vi "HighEnd-RT.vi"() -> ()   [LabVIEW 2016]
uses:
  <vilib>/rvi/interface/nirviReadWriteControl/nirviReadWriteControl.xnode
  <vilib>/rvi/interface/nirviOpenFPGA/nirviOpenFPGA.xnode
  Common-Control/Beamline sections/High Energy End/HighEnd-FPGA.vi
  Glassman Control.ctl
  GP307 cluster.ctl
  NiFpgaLv.dll
  <vilib>/Utility/error.llb/Error Cluster From Error Code.vi
  <vilib>/rvi/errors/niLvFpgaAdjustHostInterfaceError.vi
  Controls/GV states.ctl
  Controls/Faraday cup states.ctl
  <vilib>/NI_Real-Time Target Support.lvlib
  FPGA Bitfiles/PRIMEControl2017_FPGATarget3_HighEnd-FPGA_o8tZdM+PVqs.lvbitx
  <vilib>/FPGAPlugInAG/cRIO-9074/niLvFpga_Open_cRIO-9074.vi
panel:
  in  "Tab Control":T1(tab)
  out "ES Quad A+ I readback":fxp<+/-,16,5>
  out "ES Quad A+ V readback":fxp<+/-,16,5>
  out "ES Quad A- I readback":fxp<+/-,16,5>
  out "ES Quad A- V readback":fxp<+/-,16,5>
  out "ES Quad B+ I readback":fxp<+/-,16,5>
  out "Y1- Steerer V set":dbl
  out "Y2+ Steerer V set":dbl
  out "Y2- Steerer V set":dbl
  out "ES Quad A V set":dbl
  out "ES Quad B V set":dbl
  out "ES Quad B+ V readback":fxp<+/-,16,5>
  out "ES Quad B- I readback":fxp<+/-,16,5>
  out "ES Quad B- V readback":fxp<+/-,16,5>
  out "X+ Steerer I readback":fxp<+/-,26,5>
  out "X+ Steerer V readback":fxp<+/-,26,7>
  out "X- Steerer  I readback":fxp<+/-,16,5>
  out "X- Steerer V readback":fxp<+/-,16,5>
  out "Y1+ Steerer  I readback":fxp<+/-,16,5>
  out "Y1+ Steerer V readback":fxp<+/-,16,5>
  out "Y1- Steerer  I readback":fxp<+/-,16,5>
  out "Y1- Steerer V readback":fxp<+/-,16,5>
  out "Y2+ Steerer  I readback":fxp<+/-,16,5>
  out "Y2+ Steerer V readback":fxp<+/-,16,5>
  out "Y2- Steerer  I readback":fxp<+/-,16,5>
  out "Y2- Steerer V readback":fxp<+/-,16,5>
  out "X+ Steerer V set":dbl
  out "X- Steerer V set":dbl
  out "X- Steerer HV Enable":bool
  out "Y1+ Steerer V set":dbl
  out "Y1+ Steerer HV Enable":bool
  out "Y1- Steerer HV Enable":bool
  out "Y2+ Steerer HV Enable":bool
  out "Y2- Steerer HV Enable":bool
  out "ES Quad A HV Enable":bool
  out "ES Quad B HV Enable":bool
  out "X+ Steerer HV Enable":bool
  out "Analyzer Object Vac cluster":T2
  out "Tank Exit Vac cluster":T2
  out "Vac readback loop error":errorcluster
  out "Ion gauge 1":u8[](array[numeric])
  out "Convectron 1":u8[](array[numeric])
  out "Ion gauge 2":u8[](array[numeric])
  out "Convectron 2":u8[](array[numeric])
  out "Ion gauge 3":u8[](array[numeric])
  out "Convectron 4":u8[](array[numeric])
  out "Ion gauge 4":u8[](array[numeric])
  out "Convectron 4":u8[](array[numeric])
  out "High End waist interlock bypass":bool
  out "Tank Exit Vac Interlock":bool
  out "High End Waist Vac Interlock":bool
  out "Analyzer Image Vac Interlock":bool
  out "Tank Exit interlock bypass":bool
  out "Analyzer Image Interlock Bypass":bool
  out "Tank Exit FC Actuator":bool
  out "Cryo Pump GV Actuator":bool
  out "Beamline GV Actuator":bool
  out "Beamline Fast GV actuator":bool
  out "Turbo GV actuator":bool
  out "Beamline Fast GV status":T3
  out "Beamline Fast GV Position":T4
  out "Turbo GV status":T3
  out "Turbo GV Position":T4
  out "Beamline GV status":T3
  out "Beamline GV Position":T4
  out "Tank Exit FC Status":T5
  out "Tank Exit FC Position":cluster{"IN sensor":bool, "OUT sensor":bool}
  out "Cryo Pump GV status":T3
  out "Cryo Pump GV Position":T4
  out "HV readback loop error":errorcluster
  out "Interlock loop error":errorcluster
  out "Actuator Sensor loop error":errorcluster
  out "HV control loop error":errorcluster
  out "Error Reporter":errorcluster
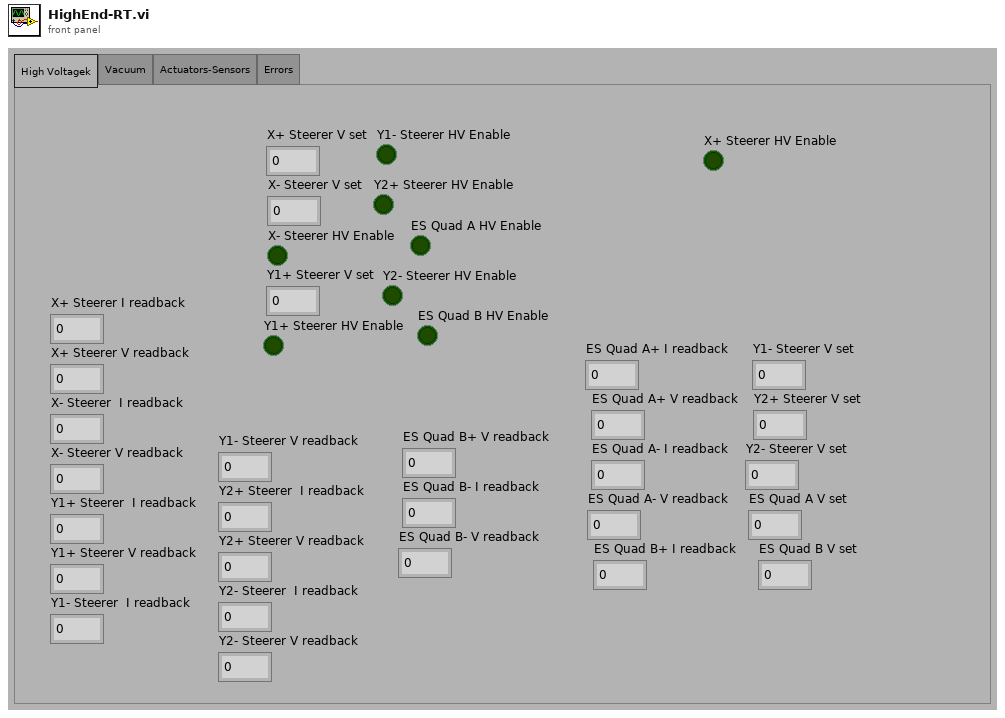
[diagram p1: front panel]
types:
  T1 = enum32{"High Voltagek", "Vacuum", "Actuators-Sensors", "Errors"}
  T2 = cluster{"Ion gauge 1":string, "Convectron  Gauge 1 ":string, "Ion Gauge 2":string, "Convectrom Gauge 2":string}
  T3 = typedef "GV states.ctl" = enum16{"status unclear", "closed", "open"}
  T4 = cluster{"OPEN sensor":bool, "Closed sensor":bool}
  T5 = typedef "Faraday cup states.ctl" = enum16{"FC status unclear", "FC in", "FC out"}
  T6 = typedef "Glassman Control.ctl" = cluster{"V-program":fxp<+/-,16,5>, "HV Enable":bool}
  T7 = typedef "GP307 cluster.ctl" = cluster{"Ion gauge 1":string, "Convectron  Gauge 1 ":string, "Ion Gauge 2":string, "Convectrom Gauge 2":string}
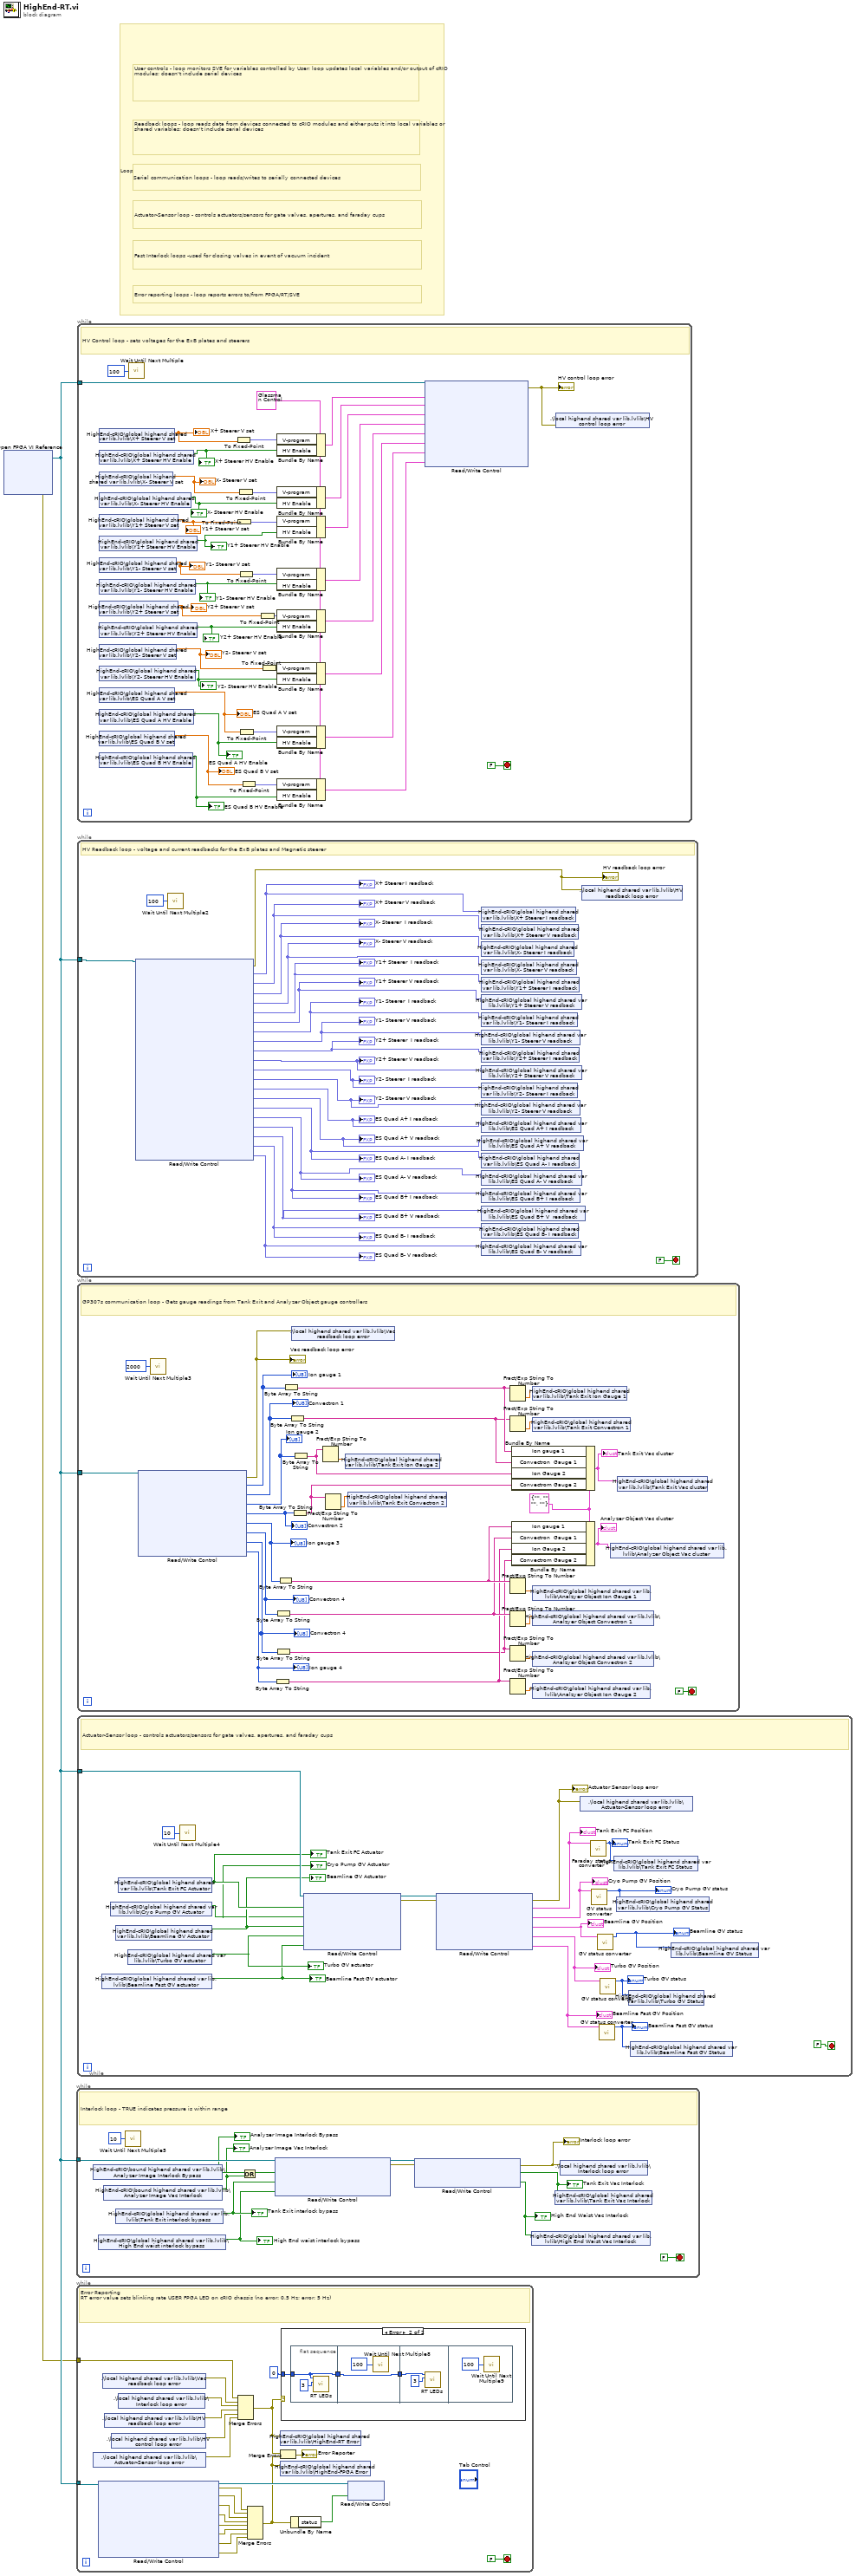
[diagram p0: block diagram]
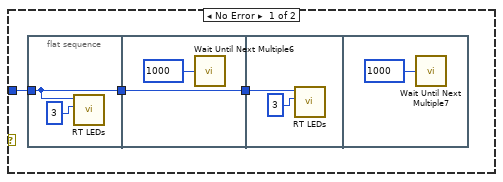
[diagram p2: hidden frame]
diagram:
  # "Serial communication loops - loop reads/writes to serially connected devices"
  # "Actuator-Sensor loop - controls actuators/sensors for gate valves, apertures, and faraday cups"
  # "Fast Interlock loops -used for closing valves in event of vacuum incident"
  # "Error reporting loops - loop reports errors to/from FPGA/RT/SVE"
  # "Readback loops - loop reads data from devices connected to cRIO modules and either puts it into local variables or shared variables; doesn't include serial devices"
  # "User controls - loop monitors SVE for variables controlled by User; loop updates local variables and/or output of cRIO modules; doesn't include serial devices"
  # "Loop legend - loops are color coded by responsibility"
  n1 = xnode "Open FPGA VI Reference"() -> ("FPGA VI Reference Out"=w2:refnum<k20>, "error out"=w1:errorcluster)  [unwired: 2 in]
  n2 = while {
    tunnel: w2 -> [w15]
    stop <- FALSE stop-if-true
    # "Interlock loop - TRUE indicates pressure is within range"
    n3 = shared-variable "HighEnd-cRIO\\bound highend shared var lib.lvlib\\Analyzer Image Interlock Bypass"() -> (w11:bool)  [unwired: 1 in, 1 out]
    "Analyzer Image Interlock Bypass" <- w11
    n4 = shared-variable "HighEnd-cRIO\\global highend shared var lib.lvlib\\High End waist interlock bypass"() -> (w6:bool)  [unwired: 1 in, 1 out]
    "High End waist interlock bypass" <- w6
    n5 = shared-variable "HighEnd-cRIO\\bound highend shared var lib.lvlib\\Analyzer Image Vac Interlock"() -> (w9:bool)  [unwired: 1 in, 1 out]
    "Analyzer Image Vac Interlock" <- w9
    n6 = shared-variable "HighEnd-cRIO\\global highend shared var lib.lvlib\\Tank Exit interlock bypass"() -> (w7:bool)  [unwired: 1 in, 1 out]
    "Tank Exit interlock bypass" <- w7
    n7 = call "Wait Until Next Multiple5"("Count(mSec)"=u32 10 ("millisecond multiple")) -> ()  [unwired: 1 out]
    n8 = Or(x=w11, y=w9) -> (x .or. y?=w10:bool)
    n9 = xnode "Read/Write Control"("FPGA VI Reference In"=w15, "Analyzer Image Vac Interlock"=w10, "Tank Exit interlock bypass"=w7, "High End waist interlock bypass"=w6) -> ("FPGA VI Reference Out"=w13:refnum<k20>, "error out"=w12:errorcluster)  [unwired: 1 in]
    n10 = xnode "Read/Write Control"("FPGA VI Reference In"=w13, "error in"=w12) -> ("error out"=w8:errorcluster, "Tank Exit Vac Interlock"=w5:bool, "High End Waist Vac Interlock"=w4:bool)  [unwired: 1 out]
    "Interlock loop error" <- w8
    "Tank Exit Vac Interlock" <- w5
    "High End Waist Vac Interlock" <- w4
    n11 = shared-variable "HighEnd-cRIO\\global highend shared var lib.lvlib\\High End Waist Vac Interlock"(w4) -> ()  [unwired: 1 in, 1 out]
    n12 = shared-variable "HighEnd-cRIO\\global highend shared var lib.lvlib\\Tank Exit Vac Interlock"(w5) -> ()  [unwired: 1 in, 1 out]
    n13 = shared-variable ".\\local highend shared var lib.lvlib\\Interlock loop error"(w8) -> ()  [unwired: 1 in, 1 out]
  }
  n14 = while {
    tunnel: w2 -> [w36]
    tunnel: w1 -> [w20]
    stop <- FALSE stop-if-true
    # "Error Reporting\nRT error value sets blinking rate USER FPGA LED on cRIO chassis (no error: 0.5 Hz; error: 5 Hz)"
    n15 = shared-variable ".\\local highend shared var lib.lvlib\\Actuator-Sensor loop error"() -> (w25:errorcluster)  [unwired: 1 in, 1 out]
    n16 = xnode "Read/Write Control"("FPGA VI Reference In"=w36) -> ("FPGA VI Reference Out"=w35:refnum<k20>, "error out"=w34:errorcluster, "GV Interlock loop error"=w33:errorcluster, "Actuator loop error"=w32:errorcluster, "Tank Exit Vac Gauge error"=w31:errorcluster, "Analyzer Obj Vac Gauge error"=w30:errorcluster, "Steerer HV readback loop error"=w29:errorcluster, "ES Quad HV readback loop error"=w28:errorcluster, "HV control loop error"=w27:errorcluster)  [unwired: 1 in]
    n17 = shared-variable ".\\local highend shared var lib.lvlib\\Vac readback loop error"() -> (w21:errorcluster)  [unwired: 1 in, 1 out]
    n18 = shared-variable ".\\local highend shared var lib.lvlib\\HV readback loop error"() -> (w23:errorcluster)  [unwired: 1 in, 1 out]
    n19 = shared-variable ".\\local highend shared var lib.lvlib\\HV control loop error"() -> (w24:errorcluster)  [unwired: 1 in, 1 out]
    n20 = shared-variable ".\\local highend shared var lib.lvlib\\Interlock loop error"() -> (w22:errorcluster)  [unwired: 1 in, 1 out]
    n21 = Merge Errors(w20, w21, w22, w23, w24, w25) -> (w16:errorcluster)
    n22 = Merge Errors(w34, w33, w32, w31, w30, w29, w28, w27) -> (w18:errorcluster)
    n23 = shared-variable "HighEnd-cRIO\\global highend shared var lib.lvlib\\HighEnd-RT Error"(w16) -> ()  [unwired: 1 in, 1 out]
    n24 = Merge Errors(w16, w18) -> (→"Error Reporter":errorcluster)
    n25 = shared-variable "HighEnd-cRIO\\global highend shared var lib.lvlib\\HighEnd-FPGA Error"(w18) -> ()  [unwired: 1 in, 1 out]
    n26 = case shown="Error" w16 {
      tunnel: 0 -> [w40 w48]
      frame No Error {
        n27 = flat-sequence {
          tunnel: w40 -> [w41]
          tunnel: [w41] -> w38
          tunnel: [w43] -> w39
          tunnel: w38 -> [w43]
          tunnel: w39 -> [w45]
          frame #0 {
            n28 = call <vilib>:"RT LEDs.vi"("State"=3, "LED Num"=w41) -> ()  [unwired: 4 in, 2 out]
          }
          frame #1 {
            n29 = call "Wait Until Next Multiple6"("Count(mSec)"=u16 1000) -> ()  [unwired: 1 out]
          }
          frame #2 {
            n30 = call <vilib>:"RT LEDs.vi"("State"=3, "LED Num"=w45) -> ()  [unwired: 4 in, 2 out]
          }
          frame #3 {
            n31 = call "Wait Until Next Multiple7"("Count(mSec)"=u16 1000) -> ()  [unwired: 1 out]
          }
        }
      }
      frame Error {
        n32 = flat-sequence {
          tunnel: [w51] -> w50
          tunnel: w48 -> [w51]
          tunnel: w50 -> [w53]
          tunnel: [w53] -> w49
          tunnel: w49 -> [w55]
          frame #0 {
            n33 = call <vilib>:"RT LEDs.vi"("State"=3, "LED Num"=w51) -> ()  [unwired: 4 in, 2 out]
          }
          frame #1 {
            n34 = call "Wait Until Next Multiple8"("Count(mSec)"=u16 100) -> ()  [unwired: 1 out]
          }
          frame #2 {
            n35 = call <vilib>:"RT LEDs.vi"("State"=3, "LED Num"=w55) -> ()  [unwired: 4 in, 2 out]
          }
          frame #3 {
            n36 = call "Wait Until Next Multiple9"("Count(mSec)"=u16 100) -> ()  [unwired: 1 out]
          }
        }
      }
    }
    n37 = Unbundle By Name(w18) -> ("status"=w37:bool)
    n38 = xnode "Read/Write Control"("FPGA VI Reference In"=w35, "RT error"=w37) -> ()  [unwired: 1 in, 2 out]
  }
  n39 = while {
    tunnel: w2 -> [w94]
    stop <- FALSE stop-if-true
    w69 = T6 {"V-program"=0.0, "HV Enable"=FALSE} ("Glassman Control")
    # "HV Control loop - sets voltages for the ExB plates and steerers"
    n40 = shared-variable "HighEnd-cRIO\\global highend shared var lib.lvlib\\X+ Steerer V set"() -> (w90:dbl)  [unwired: 1 in, 1 out]
    "X+ Steerer V set" <- w90
    n41 = shared-variable "HighEnd-cRIO\\global highend shared var lib.lvlib\\X+ Steerer HV Enable"() -> (w89:bool)  [unwired: 1 in, 1 out]
    "X+ Steerer HV Enable" <- w89
    n42 = shared-variable "HighEnd-cRIO\\global highend shared var lib.lvlib\\X- Steerer V set"() -> (w88:dbl)  [unwired: 1 in, 1 out]
    "X- Steerer V set" <- w88
    n43 = shared-variable "HighEnd-cRIO\\global highend shared var lib.lvlib\\X- Steerer HV Enable"() -> (w87:bool)  [unwired: 1 in, 1 out]
    "X- Steerer HV Enable" <- w87
    n44 = shared-variable "HighEnd-cRIO\\global highend shared var lib.lvlib\\Y1+ Steerer V set"() -> (w84:dbl)  [unwired: 1 in, 1 out]
    "Y1+ Steerer V set" <- w84
    n45 = shared-variable "HighEnd-cRIO\\global highend shared var lib.lvlib\\Y1+ Steerer HV Enable"() -> (w61:bool)  [unwired: 1 in, 1 out]
    "Y1+ Steerer HV Enable" <- w61
    n46 = shared-variable "HighEnd-cRIO\\global highend shared var lib.lvlib\\Y1- Steerer V set"() -> (w83:dbl)  [unwired: 1 in, 1 out]
    "Y1- Steerer V set" <- w83
    n47 = shared-variable "HighEnd-cRIO\\global highend shared var lib.lvlib\\Y1- Steerer HV Enable"() -> (w82:bool)  [unwired: 1 in, 1 out]
    "Y1- Steerer HV Enable" <- w82
    n48 = shared-variable "HighEnd-cRIO\\global highend shared var lib.lvlib\\Y2+ Steerer V set"() -> (w79:dbl)  [unwired: 1 in, 1 out]
    "Y2+ Steerer V set" <- w79
    n49 = shared-variable "HighEnd-cRIO\\global highend shared var lib.lvlib\\Y2+ Steerer HV Enable"() -> (w78:bool)  [unwired: 1 in, 1 out]
    "Y2+ Steerer HV Enable" <- w78
    n50 = shared-variable "HighEnd-cRIO\\global highend shared var lib.lvlib\\Y2- Steerer V set"() -> (w77:dbl)  [unwired: 1 in, 1 out]
    "Y2- Steerer V set" <- w77
    n51 = shared-variable "HighEnd-cRIO\\global highend shared var lib.lvlib\\Y2- Steerer HV Enable"() -> (w76:bool)  [unwired: 1 in, 1 out]
    "Y2- Steerer HV Enable" <- w76
    n52 = shared-variable "HighEnd-cRIO\\global highend shared var lib.lvlib\\ES Quad A V set"() -> (w73:dbl)  [unwired: 1 in, 1 out]
    "ES Quad A V set" <- w73
    n53 = shared-variable "HighEnd-cRIO\\global highend shared var lib.lvlib\\ES Quad A HV Enable"() -> (w72:bool)  [unwired: 1 in, 1 out]
    "ES Quad A HV Enable" <- w72
    n54 = shared-variable "HighEnd-cRIO\\global highend shared var lib.lvlib\\ES Quad B V set"() -> (w71:dbl)  [unwired: 1 in, 1 out]
    "ES Quad B V set" <- w71
    n55 = shared-variable "HighEnd-cRIO\\global highend shared var lib.lvlib\\ES Quad B HV Enable"() -> (w70:bool)  [unwired: 1 in, 1 out]
    "ES Quad B HV Enable" <- w70
    n56 = call "Wait Until Next Multiple"("Count(mSec)"=u32 100 ("millisecond multiple")) -> ()  [unwired: 1 out]
    n57 = To Fixed-Point(number=w90) -> (fixed-point=w58:fxp<+/-,16,5>)  [unwired: 1 in]
    n58 = To Fixed-Point(number=w84) -> (fixed-point=w86:fxp<+/-,16,5>)  [unwired: 1 in]
    n59 = To Fixed-Point(number=w88) -> (fixed-point=w92:fxp<+/-,16,5>)  [unwired: 1 in]
    n60 = To Fixed-Point(number=w83) -> (fixed-point=w85:fxp<+/-,16,5>)  [unwired: 1 in]
    n61 = To Fixed-Point(number=w73) -> (fixed-point=w75:fxp<+/-,16,5>)  [unwired: 1 in]
    n62 = To Fixed-Point(number=w71) -> (fixed-point=w74:fxp<+/-,16,5>)  [unwired: 1 in]
    n63 = To Fixed-Point(number=w79) -> (fixed-point=w81:fxp<+/-,16,5>)  [unwired: 1 in]
    n64 = To Fixed-Point(number=w77) -> (fixed-point=w80:fxp<+/-,16,5>)  [unwired: 1 in]
    n65 = Bundle By Name(cluster=w69, "V-program"=w58, "HV Enable"=w89) -> (w93:T6)
    n66 = Bundle By Name(cluster=w69, "V-program"=w92, "HV Enable"=w87) -> (w68:T6)
    n67 = Bundle By Name(cluster=w69, "V-program"=w86, "HV Enable"=w61) -> (w67:T6)
    n68 = Bundle By Name(cluster=w69, "V-program"=w85, "HV Enable"=w82) -> (w66:T6)
    n69 = Bundle By Name(cluster=w69, "V-program"=w81, "HV Enable"=w78) -> (w65:T6)
    n70 = Bundle By Name(cluster=w69, "V-program"=w80, "HV Enable"=w76) -> (w64:T6)
    n71 = Bundle By Name(cluster=w69, "V-program"=w75, "HV Enable"=w72) -> (w63:T6)
    n72 = Bundle By Name(cluster=w69, "V-program"=w74, "HV Enable"=w70) -> (w62:T6)
    n73 = xnode "Read/Write Control"("FPGA VI Reference In"=w94, "X+ Steerer V set"=w93, "X- Steerer V set"=w68, "Y1+ Steerer V set"=w67, "Y1- Steerer V set"=w66, "Y2+ Steerer V set"=w65, "Y2- Steerer V set"=w64, "ES Quad A V set"=w63, "ES Quad B V set"=w62) -> ("error out"=w60:errorcluster)  [unwired: 1 in, 1 out]
    "HV control loop error" <- w60
    n74 = shared-variable ".\\local highend shared var lib.lvlib\\HV control loop error"(error in=w60) -> ()  [unwired: 2 out]
  }
  n75 = while {
    tunnel: w2 -> [w116]
    stop <- FALSE stop-if-true
    # "HV Readback loop - voltage and current readbacks for the ExB plates and Magnetic steerer"
    n76 = xnode "Read/Write Control"("FPGA VI Reference In"=w116) -> ("error out"=w118:errorcluster, "X+ Steerer readback.I-monitor"=w115:fxp<+/-,16,5>, "X+ Steerer readback.V-monitor"=w114:fxp<+/-,16,5>, "X- Steerer readback.I-monitor"=w113:fxp<+/-,16,5>, "X- Steerer readback.V-monitor"=w112:fxp<+/-,16,5>, "Y1+ Steerer readback.I-monitor"=w111:fxp<+/-,16,5>, "Y1+ Steerer readback.V-monitor"=w110:fxp<+/-,16,5>, "Y1- Steerer readback.I-monitor"=w109:fxp<+/-,16,5>, "Y1- Steerer readback.V-monitor"=w108:fxp<+/-,16,5>, "Y2+ Steerer readback.I-monitor"=w107:fxp<+/-,16,5>, "Y2+ Steerer readback.V-monitor"=w106:fxp<+/-,16,5>, "Y2- Steerer readback.I-monitor"=w105:fxp<+/-,16,5>, "Y2- Steerer readback.V-monitor"=w104:fxp<+/-,16,5>, "ES Quad A+ readback.I-monitor"=w103:fxp<+/-,16,5>, "ES Quad A+ readback.V-monitor"=w102:fxp<+/-,16,5>, "ES Quad A- readback.I-monitor"=w96:fxp<+/-,16,5>, "ES Quad A- readback.V-monitor"=w97:fxp<+/-,16,5>, "ES Quad B+ readback.I-monitor"=w98:fxp<+/-,16,5>, "ES Quad B+ readback.V-monitor"=w99:fxp<+/-,16,5>, "ES Quad B- readback.I-monitor"=w100:fxp<+/-,16,5>, "ES Quad B- readback.V-monitor"=w101:fxp<+/-,16,5>)  [unwired: 1 in, 1 out]
    "HV readback loop error" <- w118
    "X+ Steerer I readback" <- w115
    "X+ Steerer V readback" <- w114
    "X- Steerer  I readback" <- w113
    "X- Steerer V readback" <- w112
    "Y1+ Steerer  I readback" <- w111
    "Y1+ Steerer V readback" <- w110
    "Y1- Steerer  I readback" <- w109
    "Y1- Steerer V readback" <- w108
    "Y2+ Steerer  I readback" <- w107
    "Y2+ Steerer V readback" <- w106
    "Y2- Steerer  I readback" <- w105
    "Y2- Steerer V readback" <- w104
    "ES Quad A+ I readback" <- w103
    "ES Quad A+ V readback" <- w102
    "ES Quad A- I readback" <- w96
    "ES Quad A- V readback" <- w97
    "ES Quad B+ I readback" <- w98
    "ES Quad B+ V readback" <- w99
    "ES Quad B- I readback" <- w100
    "ES Quad B- V readback" <- w101
    n77 = call "Wait Until Next Multiple2"("Count(mSec)"=u32 100 ("millisecond multiple")) -> ()  [unwired: 1 out]
    n78 = shared-variable "HighEnd-cRIO\\global highend shared var lib.lvlib\\X+ Steerer I readback"(w115) -> ()  [unwired: 1 in, 1 out]
    n79 = shared-variable "HighEnd-cRIO\\global highend shared var lib.lvlib\\X+ Steerer V readback"(w114) -> ()  [unwired: 1 in, 1 out]
    n80 = shared-variable "HighEnd-cRIO\\global highend shared var lib.lvlib\\X- Steerer I readback"(w113) -> ()  [unwired: 1 in, 1 out]
    n81 = shared-variable "HighEnd-cRIO\\global highend shared var lib.lvlib\\X- Steerer V readback"(w112) -> ()  [unwired: 1 in, 1 out]
    n82 = shared-variable "HighEnd-cRIO\\global highend shared var lib.lvlib\\Y1+ Steerer I readback"(w111) -> ()  [unwired: 1 in, 1 out]
    n83 = shared-variable "HighEnd-cRIO\\global highend shared var lib.lvlib\\Y1+ Steerer V readback"(w110) -> ()  [unwired: 1 in, 1 out]
    n84 = shared-variable "HighEnd-cRIO\\global highend shared var lib.lvlib\\Y1- Steerer I readback"(w109) -> ()  [unwired: 1 in, 1 out]
    n85 = shared-variable "HighEnd-cRIO\\global highend shared var lib.lvlib\\Y1- Steerer V readback"(w108) -> ()  [unwired: 1 in, 1 out]
    n86 = shared-variable "HighEnd-cRIO\\global highend shared var lib.lvlib\\Y2+ Steerer I readback"(w107) -> ()  [unwired: 1 in, 1 out]
    n87 = shared-variable "HighEnd-cRIO\\global highend shared var lib.lvlib\\Y2+ Steerer V readback"(w106) -> ()  [unwired: 1 in, 1 out]
    n88 = shared-variable "HighEnd-cRIO\\global highend shared var lib.lvlib\\Y2- Steerer I readback"(w105) -> ()  [unwired: 1 in, 1 out]
    n89 = shared-variable "HighEnd-cRIO\\global highend shared var lib.lvlib\\Y2- Steerer V readback"(w104) -> ()  [unwired: 1 in, 1 out]
    n90 = shared-variable "HighEnd-cRIO\\global highend shared var lib.lvlib\\ES Quad A+ I readback"(w103) -> ()  [unwired: 1 in, 1 out]
    n91 = shared-variable "HighEnd-cRIO\\global highend shared var lib.lvlib\\ES Quad A+ V readback"(w102) -> ()  [unwired: 1 in, 1 out]
    n92 = shared-variable "HighEnd-cRIO\\global highend shared var lib.lvlib\\ES Quad A- I readback"(w96) -> ()  [unwired: 1 in, 1 out]
    n93 = shared-variable "HighEnd-cRIO\\global highend shared var lib.lvlib\\ES Quad A- V readback"(w97) -> ()  [unwired: 1 in, 1 out]
    n94 = shared-variable "HighEnd-cRIO\\global highend shared var lib.lvlib\\ES Quad B+ I readback"(w98) -> ()  [unwired: 1 in, 1 out]
    n95 = shared-variable "HighEnd-cRIO\\global highend shared var lib.lvlib\\ES Quad B+ V  readback"(w99) -> ()  [unwired: 1 in, 1 out]
    n96 = shared-variable "HighEnd-cRIO\\global highend shared var lib.lvlib\\ES Quad B- I readback"(w100) -> ()  [unwired: 1 in, 1 out]
    n97 = shared-variable "HighEnd-cRIO\\global highend shared var lib.lvlib\\ES Quad B- V readback"(w101) -> ()  [unwired: 1 in, 1 out]
    n98 = shared-variable ".\\local highend shared var lib.lvlib\\HV readback loop error"(w118) -> ()  [unwired: 1 in, 1 out]
  }
  n99 = while {
    tunnel: w2 -> [w131]
    stop <- FALSE stop-if-true
    w130 = T7 {"Ion gauge 1"="", "Convectron  Gauge 1 "="", "Ion Gauge 2"="", "Convectrom Gauge 2"=""} ("Ion gauge cluster control")
    # "GP307s communication loop - Gets gauge readings from Tank Exit and Analyzer Object gauge controllers"
    n100 = xnode "Read/Write Control"("FPGA VI Reference In"=w131) -> ("error out"=w129:errorcluster, "Tank Exit Ion Gauge 1"=w146:u8[], "Tank Exit Convectron 1"=w147:u8[], "Tank Exit Ion Gauge 2"=w148:u8[], "Tank Exit Convectron 2"=w149:u8[], "Analyzer Object Ion Gauge 1"=w144:u8[], "Analyzer Object Convectron 1"=w143:u8[], "Analyzer Object Convectron 2"=w141:u8[], "Analyzer Object Ion Gauge 2"=w142:u8[])  [unwired: 1 in, 1 out]
    "Vac readback loop error" <- w129
    "Ion gauge 1" <- w146
    "Convectron 1" <- w147
    "Ion gauge 2" <- w148
    "Convectron 2" <- w149
    "Ion gauge 3" <- w144
    "Convectron 4" <- w143
    "Ion gauge 4" <- w142
    "Convectron 4" <- w141
    n101 = call "Wait Until Next Multiple3"("Count(mSec)"=u32 2000 ("millisecond multiple")) -> ()  [unwired: 1 out]
    n102 = Byte Array To String(unsigned byte array=w142) -> (string=w137:string)
    n103 = Byte Array To String(unsigned byte array=w143) -> (string=w138:string)
    n104 = Byte Array To String(unsigned byte array=w141) -> (string=w136:string)
    n105 = Byte Array To String(unsigned byte array=w144) -> (string=w139:string)
    n106 = Byte Array To String(unsigned byte array=w146) -> (string=w135:string)
    n107 = Byte Array To String(unsigned byte array=w147) -> (string=w134:string)
    n108 = shared-variable ".\\local highend shared var lib.lvlib\\Vac readback loop error"(w129) -> ()  [unwired: 1 in, 1 out]
    n109 = Byte Array To String(unsigned byte array=w149) -> (string=w132:string)
    n110 = Byte Array To String(unsigned byte array=w148) -> (string=w133:string)
    n111 = Fract/Exp String To Number(string=w133) -> (number=w128:dbl)  [unwired: 3 in, 1 out]
    n112 = Fract/Exp String To Number(string=w132) -> (number=w127:dbl)  [unwired: 3 in, 1 out]
    n113 = shared-variable "HighEnd-cRIO\\global highend shared var lib.lvlib\\Tank Exit Ion Gauge 2"(w128) -> ()  [unwired: 1 in, 1 out]
    n114 = shared-variable "HighEnd-cRIO\\global highend shared var lib.lvlib\\Tank Exit Convectron 2"(w127) -> ()  [unwired: 1 in, 1 out]
    n115 = Fract/Exp String To Number(string=w135) -> (number=w126:dbl)  [unwired: 3 in, 1 out]
    n116 = Fract/Exp String To Number(string=w134) -> (number=w125:dbl)  [unwired: 3 in, 1 out]
    n117 = Fract/Exp String To Number(string=w139) -> (number=w124:dbl)  [unwired: 3 in, 1 out]
    n118 = Fract/Exp String To Number(string=w138) -> (number=w123:dbl)  [unwired: 3 in, 1 out]
    n119 = Fract/Exp String To Number(string=w136) -> (number=w122:dbl)  [unwired: 3 in, 1 out]
    n120 = Fract/Exp String To Number(string=w137) -> (number=w121:dbl)  [unwired: 3 in, 1 out]
    n121 = Bundle By Name(cluster=w130, "Ion gauge 1"=w135, "Convectron  Gauge 1"=w134, "Ion Gauge 2"=w133, "Convectrom Gauge 2"=w132) -> (w140:T7)
    "Tank Exit Vac cluster" <- w140
    n122 = Bundle By Name(cluster=w130, "Ion gauge 1"=w139, "Convectron  Gauge 1"=w138, "Ion Gauge 2"=w137, "Convectrom Gauge 2"=w136) -> (w120:T7)
    "Analyzer Object Vac cluster" <- w120
    n123 = shared-variable "HighEnd-cRIO\\global highend shared var lib.lvlib\\Tank Exit Ion Gauge 1"(w126) -> ()  [unwired: 1 in, 1 out]
    n124 = shared-variable "HighEnd-cRIO\\global highend shared var lib.lvlib\\Tank Exit Convectron 1"(w125) -> ()  [unwired: 1 in, 1 out]
    n125 = shared-variable "HighEnd-cRIO\\global highend shared var lib.lvlib\\Analzyer Object Ion Gauge 1"(w124) -> ()  [unwired: 1 in, 1 out]
    n126 = shared-variable "HighEnd-cRIO\\global highend shared var lib.lvlib\\Analzyer Object Convectron 1"(w123) -> ()  [unwired: 1 in, 1 out]
    n127 = shared-variable "HighEnd-cRIO\\global highend shared var lib.lvlib\\Analzyer Object Convectron 2"(w122) -> ()  [unwired: 1 in, 1 out]
    n128 = shared-variable "HighEnd-cRIO\\global highend shared var lib.lvlib\\Analzyer Object Ion Gauge 2"(w121) -> ()  [unwired: 1 in, 1 out]
    n129 = shared-variable "HighEnd-cRIO\\global highend shared var lib.lvlib\\Analyzer Object Vac cluster"(w120) -> ()  [unwired: 1 in, 1 out]
    n130 = shared-variable "HighEnd-cRIO\\global highend shared var lib.lvlib\\Tank Exit Vac cluster"(w140) -> ()  [unwired: 1 in, 1 out]
  }
  n131 = while {
    tunnel: w2 -> [w160]
    stop <- FALSE stop-if-true
    # "Actuator-Sensor loop - controls actuators/sensors for gate valves, apertures, and faraday cups"
    n132 = shared-variable "HighEnd-cRIO\\global highend shared var lib.lvlib\\Beamline Fast GV actuator"() -> (w156:bool)  [unwired: 1 in, 1 out]
    "Beamline Fast GV actuator" <- w156
    n133 = shared-variable "HighEnd-cRIO\\global highend shared var lib.lvlib\\Cryo Pump GV Actuator"() -> (w155:bool)  [unwired: 1 in, 1 out]
    "Cryo Pump GV Actuator" <- w155
    n134 = shared-variable "HighEnd-cRIO\\global highend shared var lib.lvlib\\Beamline GV Actuator"() -> (w158:bool)  [unwired: 1 in, 1 out]
    "Beamline GV Actuator" <- w158
    n135 = shared-variable "HighEnd-cRIO\\global highend shared var lib.lvlib\\Tank Exit FC Actuator"() -> (w159:bool)  [unwired: 1 in, 1 out]
    "Tank Exit FC Actuator" <- w159
    n136 = shared-variable "HighEnd-cRIO\\global highend shared var lib.lvlib\\Turbo GV actuator"() -> (w157:bool)  [unwired: 1 in, 1 out]
    "Turbo GV actuator" <- w157
    n137 = call "Wait Until Next Multiple4"("Count(mSec)"=u32 10 ("millisecond multiple")) -> ()  [unwired: 1 out]
    n138 = xnode "Read/Write Control"("FPGA VI Reference In"=w160, "Tank Exit FC Actuator"=w159, "Cryo Pump GV Actuator"=w155, "Beamline GV Actuator"=w158, "Turbo GV actuator"=w157, "Beamline Fast GV actuator"=w156) -> ("FPGA VI Reference Out"=w169:refnum<k20>, "error out"=w168:errorcluster)  [unwired: 1 in]
    n139 = xnode "Read/Write Control"("FPGA VI Reference In"=w169, "error in"=w168) -> ("error out"=w154:errorcluster, "Tank Exit FC Position"=w164:cluster{"IN sensor":bool, "OUT sensor":bool}, "Cryo Pump GV Position"=w161:T4, "Beamline GV Position"=w166:T4, "Turbo GV Position"=w163:T4, "Beamline Fast GV Position"=w165:T4)  [unwired: 1 out]
    "Actuator Sensor loop error" <- w154
    "Cryo Pump GV Position" <- w161
    "Tank Exit FC Position" <- w164
    "Beamline GV Position" <- w166
    "Turbo GV Position" <- w163
    "Beamline Fast GV Position" <- w165
    n140 = shared-variable ".\\local highend shared var lib.lvlib\\Actuator-Sensor loop error"(w154) -> ()  [unwired: 1 in, 1 out]
    n141 = call "Faraday status converter.vi"("FC Position"=w164) -> ("FC Status"=w167:T5)  [unwired: 10 in]
    "Tank Exit FC Status" <- w167
    n142 = call "GV status converter.vi"("Gate Valve"=w161) -> ("GV Status"=w162:T3)  [unwired: 10 in]
    "Cryo Pump GV status" <- w162
    n143 = call "GV status converter.vi"("Gate Valve"=w166) -> ("GV Status"=w151:T3)  [unwired: 10 in]
    "Beamline GV status" <- w151
    n144 = call "GV status converter.vi"("Gate Valve"=w165) -> ("GV Status"=w153:T3)  [unwired: 10 in]
    "Beamline Fast GV status" <- w153
    n145 = call "GV status converter.vi"("Gate Valve"=w163) -> ("GV Status"=w152:T3)  [unwired: 10 in]
    "Turbo GV status" <- w152
    n146 = shared-variable "HighEnd-cRIO\\global highend shared var lib.lvlib\\Tank Exit FC Status"(w167) -> ()  [unwired: 1 in, 1 out]
    n147 = shared-variable "HighEnd-cRIO\\global highend shared var lib.lvlib\\Cryo Pump GV Status"(w162) -> ()  [unwired: 1 in, 1 out]
    n148 = shared-variable "HighEnd-cRIO\\global highend shared var lib.lvlib\\Turbo GV Status"(w152) -> ()  [unwired: 1 in, 1 out]
    n149 = shared-variable "HighEnd-cRIO\\global highend shared var lib.lvlib\\Beamline Fast GV Status"(w153) -> ()  [unwired: 1 in, 1 out]
    n150 = shared-variable "HighEnd-cRIO\\global highend shared var lib.lvlib\\Beamline GV Status"(w151) -> ()  [unwired: 1 in, 1 out]
  }
